vi "avg 5 terms (SubVI).vi"(6 "Result":dynamicdata(waveform), 7 "Result 3":dynamicdata(waveform), 8 "error in (no error)":errorcluster, 9 "Result 4":dynamicdata(waveform), 10 "Result 5":dynamicdata(waveform), 11 "Result 2":dynamicdata(waveform)) -> (0 "error out":errorcluster, 3 "Dynamic Data":dynamicdata(waveform))   [LabVIEW 2019]
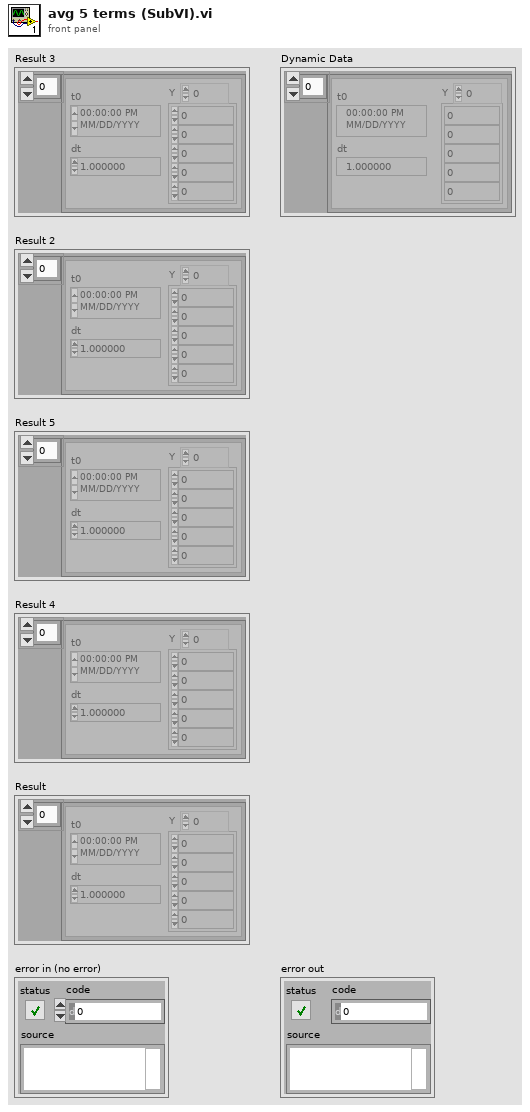
[diagram p1: front panel]
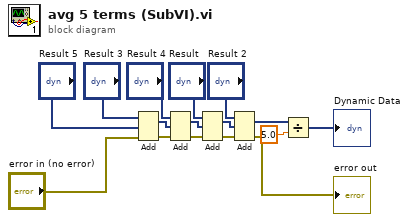
[diagram p0: block diagram]
diagram:
  n1 = Add(1:"Result 5", 2:"Result 3", 4:"error in (no error)") -> (0:w6:dynamicdata, 3:w12:errorcluster)
  n2 = Add(1:w6, 2:"Result 4", 4:w12) -> (0:w4:dynamicdata, 3:w13:errorcluster)
  n3 = Add(1:w4, 2:"Result", 4:w13) -> (0:w3:dynamicdata, 3:w14:errorcluster)
  n4 = Add(1:w3, 2:"Result 2", 4:w14) -> (0:w11:dynamicdata, 3:→"error out":errorcluster)
  n5 = Divide(x=w11, y=5.0) -> (x/y=→"Dynamic Data":dynamicdata)
